vi "Create TXT file.vi"() -> ()   [LabVIEW 2018, in "Application.lvlib"]
uses:
  Libraries/Application/Application.lvlib
panel:
  out "Array":string[](array[string])
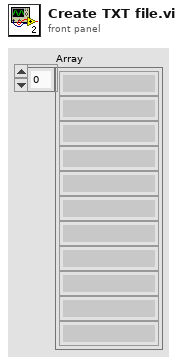
[diagram p1: front panel]
types:
  T1 = enum16{"open", "replace", "create", "open or create", "replace or create", "replace or create with confirmation"}
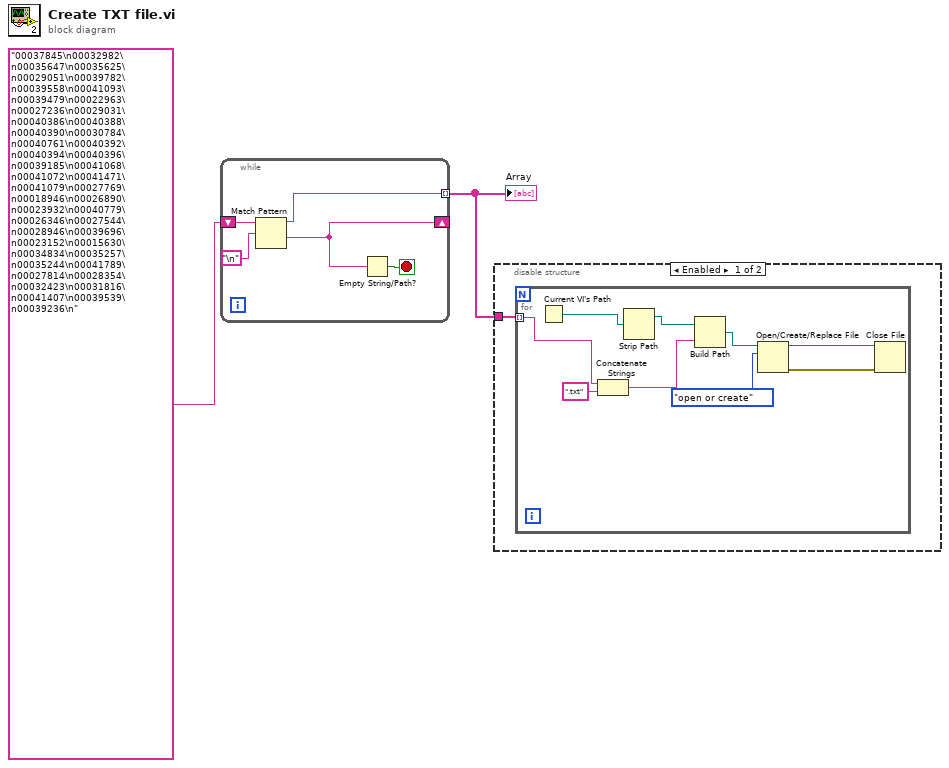
[diagram p0: block diagram]
diagram:
  n1 = while {
    shift-right: [w4] -> _
    shift-left: "00037845\n00032982\n00035647\n00035625\n00029051\n00039782\n00039558\n00041093\n00039479\n00022963\n00027236\n00029031\n00040386\n00040388\n00040390\n00030784\n00040761\n00040392\n00040394\n00040396\n00039185\n00041068\n00041072\n00041471\n00041079\n00027769\n00018946\n00026890\n00023932\n00040779\n00026346\n00027544\n00028946\n00039696\n00023152\n00015630\n00034834\n00035257\n00035244\n00041789\n00027814\n00028354\n00032423\n00031816\n00041407\n00039539\n00039236\n" -> [w7]
    tunnel: [w5] -> w1 mode=indexing
    stop <- w3 stop-if-true
    n2 = Match Pattern(string=w7, regular expression="\n") -> (before substring=w5:string, after substring=w4:string)  [unwired: 1 in, 2 out]
    n3 = Empty String/Path?(string/path=w4) -> (empty?=w3:bool)
  }
  "Array" <- w1
  n4 = disable-structure shown="Enabled" {
    disable-tunnel: w1 -> [w8 _]
    frame Enabled {
      n5 = for {
        tunnel: w8 -> [w9] mode=indexing
        n6 = Current VI's Path() -> (path=w13:path)
        n7 = Concatenate Strings(w9, ".txt" ("string")) -> (w10:string)
        n8 = Strip Path(path=w13) -> (stripped path=w12:path)  [unwired: 1 out]
        n9 = Build Path(base path=w12, name or relative path=w10) -> (appended path=w14:path)
        n10 = Open/Create/Replace File(file path (use dialog)=w14, operation (0:open)=T1."open or create") -> (refnum out=w15:refnum<file>, error out=w16:errorcluster)  [unwired: 4 in, 1 out]
        n11 = Close File(refnum=w15, error in=w16) -> ()  [unwired: 2 out]
      }
    }
    frame Disabled {
    }
  }
